vi "Excel Report.vi"() -> ()   [LabVIEW 2014]
doc: "This example shows how to generate a report from a template. The template contains a preformatted table and a preformatted graph which are updated with Append Table to Report.vi and Excel Update Graph.vi."
uses:
  <vilib>/Utility/NIReport.llb/Append Numeric Table to Report (wrap).vi
  <vilib>/Utility/NIReport.llb/NI_report.lvclass
  <vilib>/Utility/NIReport.llb/Excel/NI_Excel.lvclass
panel:
  out "transposed array":dbl[][](array[numeric])
  in  "Express VI?":bool
  in  "Test operator":string="Operator's name"
  in  "Pressure":string="100"
  in  "Humidity":string="70"
  in  "Temperature":string="20"
  in  "Data":string[][](table)=[["100", "41.7", "38.5"], ["125", "41.7", "35.2"], ["160", "41.5", "37.5"], ["200", "42.3", "42.5"], ["250", "46.9", "46.8"], ["315", "51.9", "52.6"], ["400", "52.3", "46.7"], ["500  ", "46.5", "41.6"], ["630", "42.3", "35.9"], ["800", "41.1", "32.6"]]
  # "Overview: This example shows how to generate a report from a template using either the Excel Report Generation VIs or the MS Office Report Express VI.\nRequirements: Report Generation Toolkit, Microsoft Excel\nInstructions:\nRun the VI."
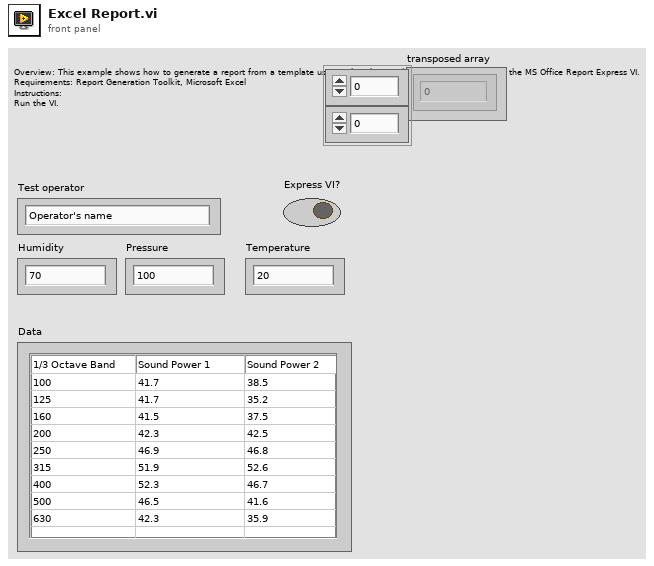
[diagram p1: front panel]
types:
  T1 = enum16{"maximized", "minimized", "normal", "no change"}
  T2 = cluster{"position (Excel)":cluster{"row":i32, "column":i32}, "name (Excel)":string, "bookmark (Word)":string}
  T3 = enum16{"Standard Report", "HTML", "Word", "Excel"}
  T4 = cluster{"position (Excel)":cluster{"row":i32, "column":i32}, "bookmark (Word)":string}
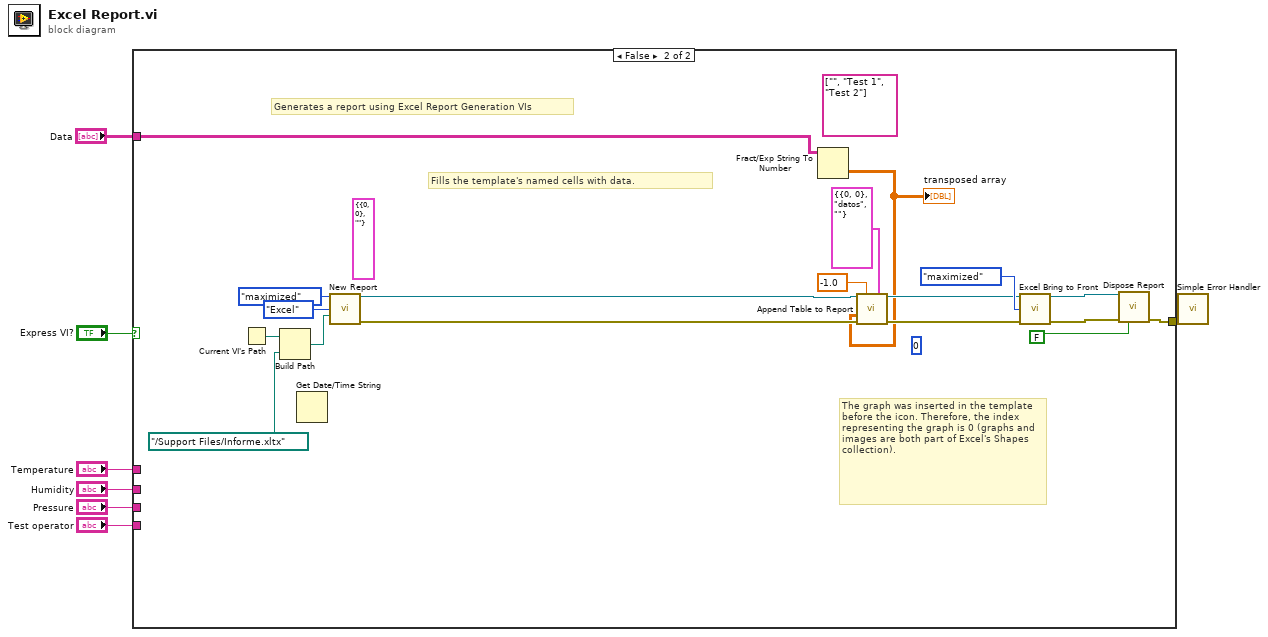
[diagram p0: block diagram]
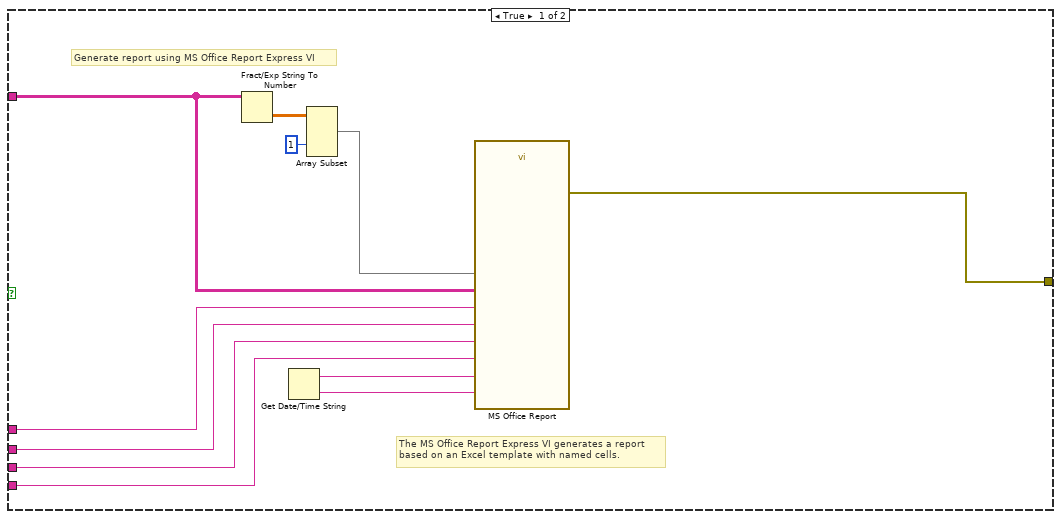
[diagram p2: hidden frame]
diagram:
  n1 = case shown="False" "Express VI?" {
    tunnel: "Temperature" -> [w13 _]
    tunnel: "Humidity" -> [w12 _]
    tunnel: "Pressure" -> [w11 _]
    tunnel: "Test operator" -> [w10 _]
    tunnel: [w14 w36] -> w3
    tunnel: "Data" -> [w15 w27]
    frame True {
      # "Generate report using MS Office Report Express VI"
      # "The MS Office Report Express VI generates a report\nbased on an Excel template with named cells."
      n2 = Fract/Exp String To Number(string=w15) -> (number=w18:dbl[][])  [unwired: 3 in, 1 out]
      n3 = Get Date/Time String() -> (date string=w9:string, time string=w8:string)  [unwired: 3 in]
      n4 = Array Subset(array=w18, index (col)=1 ("index")) -> (w16:dbl[][])  [unwired: 3 in]
      n5 = call "MS Office Report"("chart"=w16, "data"=w15, "date"=w9, "humidity"=w12, "operator"=w10, "pressure"=w11, "temperature"=w13, "time"=w8) -> ("error out"=w14:errorcluster)  [unwired: 19 in]
    }
    frame False {
      (unwired) T4 {"position (Excel)"={"row"=0, "column"=0}, "bookmark (Word)"=""} ("MS Office parameters")
      (unwired) i16 0 ("graph index")
      (unwired) string[] ["", "Test 1", "Test 2"] ("row header")
      # "Fills the template's named cells with data."
      # "The graph was inserted in the template before the icon. Therefore, the index representing the graph is 0 (graphs and images are both part of Excel's Shapes collection)."
      # "Generates a report using Excel Report Generation VIs"
      n6 = Current VI's Path() -> (path=w28:path)
      n7 = Build Path(base path=w28, name or relative path=path "../Support Files/Informe.xltx") -> (appended path=w19:path)
      n8 = Get Date/Time String() -> ()  [unwired: 3 in, 2 out]
      n9 = call <vilib>:"New Report.vi"("window state (normal)"=T1."maximized", "report type"=T3."Excel", "template (empty)"=w19) -> ("report out"=w23:refnum<class "NI_report.lvclass">, "error out"=w22:errorcluster)  [unwired: 11 in]
      n10 = Fract/Exp String To Number(string=w27) -> (number=w21:dbl[][])  [unwired: 3 in, 1 out]
      "transposed array" <- w21
      n11 = call-poly <vilib>:"Append Table to Report.vi"("report in"=w23, "column width (1)"=-1.0, "MS Office parameters"=T2 {"position (Excel)"={"row"=0, "column"=0}, "name (Excel)"="datos", "bookmark (Word)"=""}, "numerical data"=w21, "error in (no error)"=w22) -> ("report out"=w25:refnum<class "NI_report.lvclass">, "error out"=w24:errorcluster)  [unwired: 7 in, 2 out]
      n12 = call <vilib>:"Excel Bring to Front.vi"("report in"=w25, "window state (maximized)"=enum16{"maximized", "minimized", "normal"}."maximized", "error in (no error)"=w24) -> ("report out"=w33:refnum<class "NI_report.lvclass">, "error out"=w32:errorcluster)  [unwired: 11 in]
      n13 = call-dynamic "Dispose Report.vi"("report in"=w33, "error in (no error)"=w32, "close report? (T)"=FALSE ("Close Report? (T)")) -> ("error out"=w36:errorcluster)  [unwired: 12 in]
    }
  }
  n14 = call <vilib>:"Simple Error Handler.vi"("error in (no error)"=w3) -> ()  [unwired: 4 in, 5 out]
